vi "SpecificVI - Start Modal SubVI.vi"(0 "Sequence Context In":refnum<k7>, 1 "This VI":refnum<vi>) -> (2 "Sequence Context Out":refnum<k7>, 3 "Modal ID":i32, 4 "VI Originally Open":bool, 5 "error out":errorcluster)   [LabVIEW 2009]
uses:
  <vilib>/addons/TestStand/_TSUtility.llb/TestStand - Start Modal Dialog (Sequence Context).vi
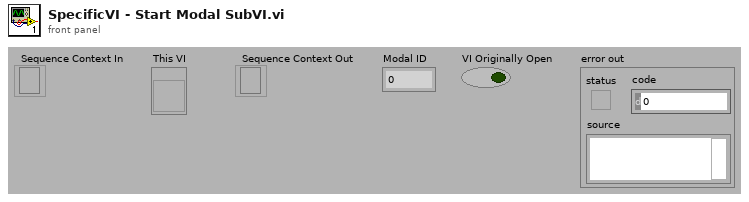
[diagram p1: front panel]
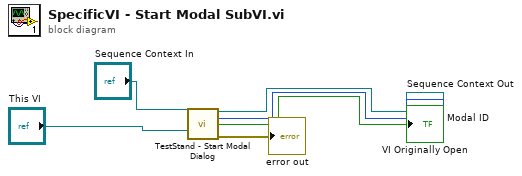
[diagram p0: block diagram]
diagram:
  n1 = call-poly <vilib>:"TestStand - Start Modal Dialog.vi"("Sequence Context In"="Sequence Context In", "VI to make Modal (Current VI)"="This VI") -> ("Sequence Context Out"=→"Sequence Context Out":refnum<k7>, "Modal ID"=→"Modal ID":i32, "VI Originally Open"=→"VI Originally Open":bool, "error out"=→"error out":errorcluster)  [unwired: 9 in, 1 out]
